vi "histogram1_cam.vi"() -> ()   [LabVIEW 2020]
uses:
  <vilib>/userdefined/High Color/IMAQdx.ctl
  <vilib>/vision/driver/NI_Vision_Acquisition_Software.lvlib
  <vilib>/vision/NI_Vision_Development_Module.lvlib
panel:
  out "히스토그램":u32[][](graph)
  in  "정지":bool
  in  "캡쳐":bool
  out "Image":T1(plugin-control)
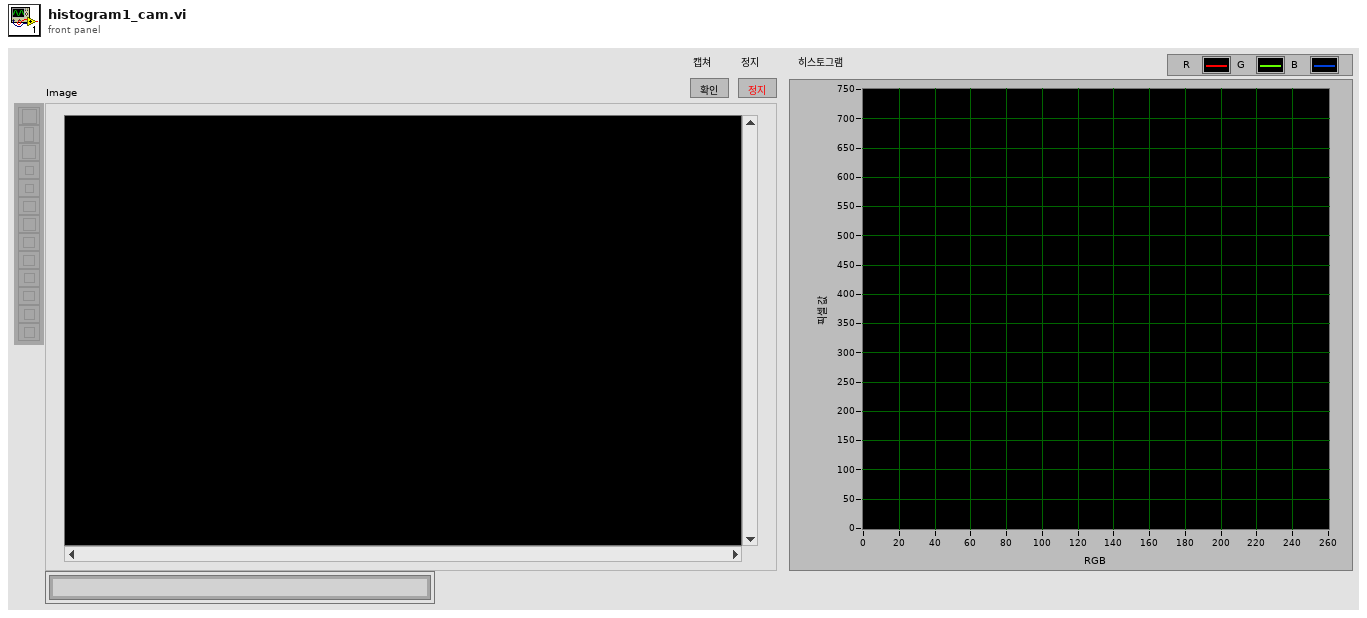
[diagram p1: front panel]
types:
  T1 = typedef "IMAQ Image.ctl" = refnum<image>
  T2 = typedef "IMAQdx.ctl" = refnum<k21>
  T3 = typedef "ROI Descriptor" = cluster{"Global Rectangle":i32[], "Contours":cluster{"ID":enum32{"External", "Internal"}, "Type":u32, "Coordinates":i32[]}[]}
  T4 = cluster{"histogram":u32[], "Minimal Value":sgl, "Maximal Value":sgl, "Starting Value":sgl, "Interval Width":sgl, "Mean Value":sgl, "Standard  Variation":sgl, "Area (pixels)":i32}
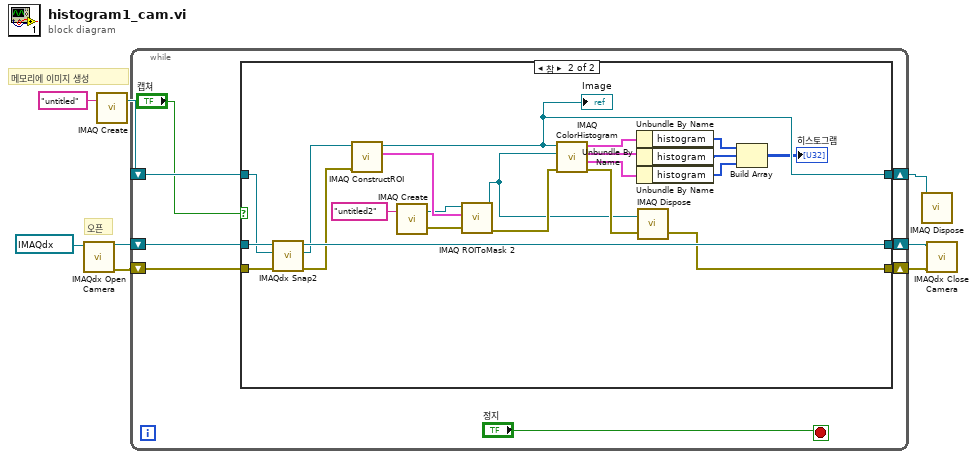
[diagram p0: block diagram]
diagram:
  # "오픈"
  # "메모리에 이미지 생성"
  n1 = call <vilib>:"IMAQdx Open Camera.vi"("Session In"=T2 "cam0") -> ("error out"=w5:errorcluster, "Session Out"=w7:T2)  [unwired: 9 in]
  n2 = call "IMAQ Create"("Image Name"="untitled") -> ("New Image"=w6:T1)  [unwired: 4 in, 1 out]
  n3 = while {
    shift-right: [w13] -> w4
    shift-left: w7 -> [w16]
    shift-right: [w11] -> w1
    shift-left: w6 -> [w15]
    shift-right: [w12] -> w3
    shift-left: w5 -> [w14]
    stop <- "정지" stop-if-true
    n4 = case shown="참" "캡쳐" {
      tunnel: w16 -> [w18 w41]
      tunnel: w15 -> [w19 w40]
      tunnel: w14 -> [w17 w39]
      tunnel: [w18 w38] -> w13
      tunnel: [w17 w30] -> w12
      tunnel: [w19 w28] -> w11
      frame False {
      }
      frame True {
        n5 = call <vilib>:"IMAQdx Snap2.vi"("error in"=w39, "Image In"=w40, "Session In"=w41) -> ("error out"=w35:errorcluster, "Image Out"=w36:T1, "Session Out"=w38:T2)  [unwired: 6 in]
        n6 = call "IMAQ ConstructROI"("error in (no error)"=w35, "Image"=w36) -> ("ROI Descriptor Out"=w34:T3, "Image Out (duplicate)"=w28:T1)  [unwired: 6 in, 2 out]
        "Image" <- w28
        n7 = call "IMAQ Create"("Image Name"="untitled2") -> ("New Image"=w21:T1, "error out"=w33:errorcluster)  [unwired: 4 in]
        n8 = call "IMAQ ROIToMask 2"("error in (no error)"=w33, "ROI Descriptor"=w34, "Image"=w21) -> ("error out"=w32:errorcluster, "Image Out"=w29:T1)  [unwired: 6 in, 1 out]
        n9 = call "IMAQ ColorHistogram"("Image Src"=w28, "Image Mask"=w29, "error in (no error)"=w32) -> ("Red or Hue or X or L* Histogram Report"=w27:T4, "Green or Sat or Y or a* Histogram Report"=w26:T4, "Blue or Luma or Val or Inten or Z or b* Histogram Report"=w25:T4, "error out"=w31:errorcluster)  [unwired: 3 in]
        n10 = Unbundle By Name(w27) -> ("histogram"=w24:u32[])
        n11 = Unbundle By Name(w26) -> ("histogram"=w23:u32[])
        n12 = Unbundle By Name(w25) -> ("histogram"=w22:u32[])
        n13 = call "IMAQ Dispose"("Image"=w29, "error in (no error)"=w31) -> ("error out"=w30:errorcluster)  [unwired: 4 in]
        n14 = Build Array(w24, w23, w22) -> (→"히스토그램":u32[][])
      }
    }
  }
  n15 = call "IMAQ Dispose"("Image"=w1) -> ()  [unwired: 5 in, 1 out]
  n16 = call <vilib>:"IMAQdx Close Camera.vi"("error in"=w3, "Session In"=w4) -> ()  [unwired: 9 in, 1 out]
